vi "ExportDataToExcel.vi"(1 "DataForAnalysis":T1(array[cluster]) {"Eff" scale=0.0..30.0}, 2 "HeaderJVMetrics":string[](array[string])=["Voc (V)", "Jsc (mA/cm2)", "FF", "P (mW/cm2)", "Hyst P1/P2", "Voc (V)", "Jsc (mA/cm2)", "FF", "P (mW/cm2)", "scan rate (mV/s)", "intensity (suns)", "temperature (C)"], 3 "title":string) -> ()   [LabVIEW 2020]
uses:
  <vilib>/Utility/NIReport.llb/NI_report.lvclass
  <vilib>/addons/_office/excel.llb/Excel Easy Table (str).vi
panel:
  # "Add a title for your excel report"
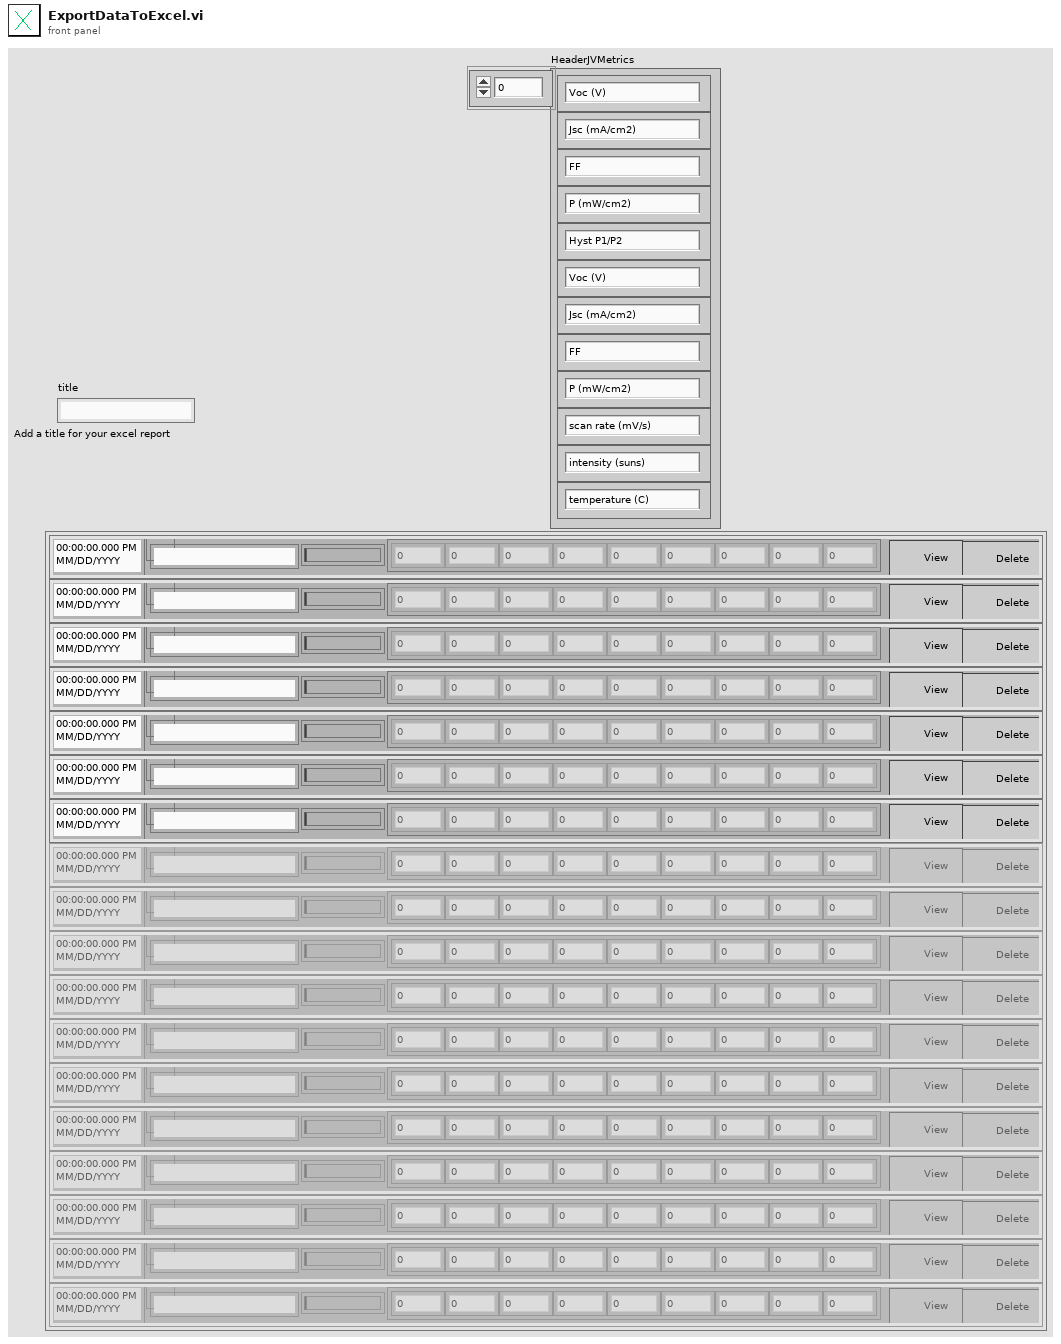
[diagram p1: front panel]
types:
  T1 = cluster{"JVData":dbl[][], "JVmetrics":dbl[], "TransientData":dbl[][], "TimeMeasured":timestamp, "Name":string, "Delete":bool, "Eff":u8, "ViewJV":bool}[]
  T2 = enum16{"Standard Report", "HTML", "Word", "Excel"}
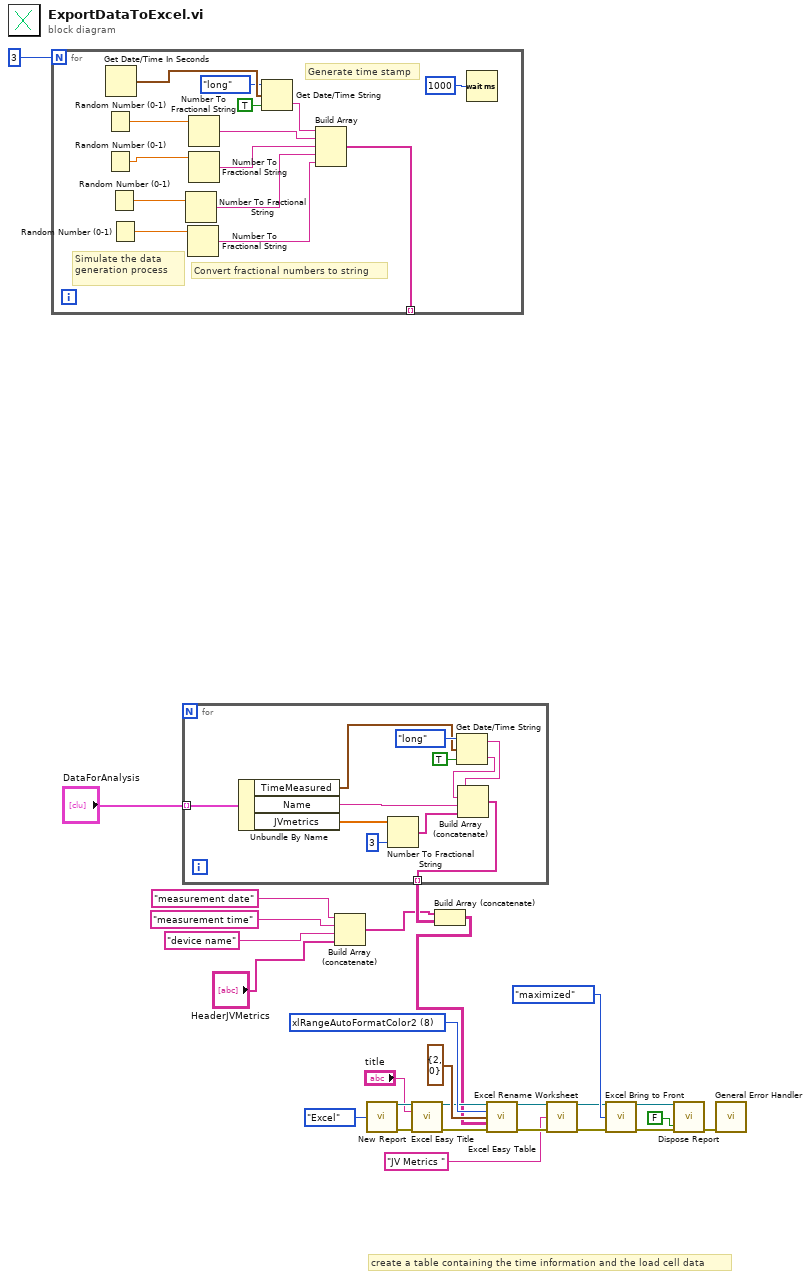
[diagram p0: block diagram]
diagram:
  w22 = 8 items=["xlRangeAutoFormat3DEffects1"=13, "xlRangeAutoFormat3DEffects2"=14, "xlRangeAutoFormatAccounting1"=4, "xlRangeAutoFormatAccounting2"=5, "xlRangeAutoFormatAccounting3"=6, "xlRangeAutoFormatAccounting4"=17, "xlRangeAutoFormatClassic1"=1, "xlRangeAutoFormatClassic2"=2, "xlRangeAutoFormatClassic3"=3, "xlRangeAutoFormatColor1"=7, "xlRangeAutoFormatColor2"=8, "xlRangeAutoFormatColor3"=9, "xlRangeAutoFormatList1"=10, "xlRangeAutoFormatList2"=11, "xlRangeAutoFormatList3"=12, "xlRangeAutoFormatLocalFormat1"=15, "xlRangeAutoFormatLocalFormat2"=16, "xlRangeAutoFormatLocalFormat3"=19, "xlRangeAutoFormatLocalFormat4"=20, "xlRangeAutoFormatReport1"=21, "xlRangeAutoFormatReport2"=22, "xlRangeAutoFormatReport3"=23, "xlRangeAutoFormatReport4"=24, "xlRangeAutoFormatReport5"=25, "xlRangeAutoFormatReport6"=26, "xlRangeAutoFormatReport7"=27, "xlRangeAutoFormatReport8"=28, "xlRangeAutoFormatReport9"=29, "xlRangeAutoFormatReport10"=30, "xlRangeAutoFormatClassicPivotTable"=31, "xlRangeAutoFormatTable1"=32, "xlRangeAutoFormatTable2"=33, "xlRangeAutoFormatTable3"=34, "xlRangeAutoFormatTable4"=35, "xlRangeAutoFormatTable5"=36, "xlRangeAutoFormatTable6"=37, "xlRangeAutoFormatTable7"=38, "xlRangeAutoFormatTable8"=39, "xlRangeAutoFormatTable9"=40, "xlRangeAutoFormatTable10"=41, "xlRangeAutoFormatPTNone"=42, "xlRangeAutoFormatNone"=-4142, "xlRangeAutoFormatSimple"=-4154] ("auto format")
  # "create a table containing the time information and the load cell data"
  n1 = for {
    N: 3 -> [_]
    tunnel: [w30] -> _ mode=indexing
    # "Convert fractional numbers to string"
    # "Generate time stamp"
    # "Simulate the data generation process"
    n2 = Random Number (0-1)() -> (number: 0 to 1=w38:dbl)
    n3 = Random Number (0-1)() -> (number: 0 to 1=w37:dbl)
    n4 = Get Date/Time In Seconds() -> (seconds since 1Jan1904=w41:timestamp)
    n5 = Random Number (0-1)() -> (number: 0 to 1=w36:dbl)
    n6 = Random Number (0-1)() -> (number: 0 to 1=w35:dbl)
    n7 = Number To Fractional String(number=w36) -> (F-format string=w32:string)  [unwired: 3 in]
    n8 = Number To Fractional String(number=w35) -> (F-format string=w31:string)  [unwired: 3 in]
    n9 = Number To Fractional String(number=w38) -> (F-format string=w34:string)  [unwired: 3 in]
    n10 = Number To Fractional String(number=w37) -> (F-format string=w33:string)  [unwired: 3 in]
    n11 = Get Date/Time String(date format (0)=enum16{"short", "long", "abbreviated"}."long", seconds (now)=w41, want seconds? (F)=TRUE) -> (time string=w28:string)  [unwired: 1 out]
    n12 = Build Array(w28, w34, w33, w32, w31) -> (w30:string[])
    n13 = Wait (ms)(milliseconds to wait=u32 1000) -> ()  [unwired: 1 out]
  }
  n14 = for {
    tunnel: "DataForAnalysis" -> [w52] mode=indexing
    tunnel: [w46] -> w12 mode=indexing
    n15 = Unbundle By Name(w52) -> ("TimeMeasured"=w47:timestamp, "Name"=w51:string, "JVmetrics"=w43:dbl[])
    n16 = Number To Fractional String(number=w43, precision (6)=i16 3) -> (F-format string=w44:string[])  [unwired: 2 in]
    n17 = Get Date/Time String(date format (0)=enum16{"short", "long", "abbreviated"}."long", seconds (now)=w47, want seconds? (F)=TRUE) -> (date string=w45:string, time string=w48:string)
    n18 = Build Array (concatenate)(w45, w48, w51, w44) -> (w46:string[])
  }
  n19 = Build Array (concatenate)("measurement date", "measurement time", "device name", "HeaderJVMetrics") -> (w8:string[])
  n20 = call <vilib>:"New Report.vi"("report type"=T2."Excel") -> ("report out"=w24:refnum<class "NI_report.lvclass">, "error out"=w25:errorcluster)  [unwired: 13 in]
  n21 = call <vilib>:"Excel Easy Title.vi"("report in"=w24, "title"="title", "error in (no error)"=w25) -> ("report out"=w16:refnum<class "NI_report.lvclass">, "error out"=w15:errorcluster)  [unwired: 10 in, 1 out]
  n22 = Build Array (concatenate)(w8, w12) -> (w7:string[][])
  n23 = call-poly <vilib>:"Excel Easy Table.vi"("report in"=w16, "auto format (none)"=w22, "start (0, 0)"=cluster{"row":i32, "column":i32} {"row"=2, "column"=0} ("position"), "text data"=w7, "error in (no error)"=w15) -> ("report out"=w5:refnum<class "NI_report.lvclass">, "error out"=w4:errorcluster)  [unwired: 6 in, 3 out]
  n24 = call <vilib>:"Excel Rename Worksheet.vi"("report in"=w5, "worksheet name (\"\")"="JV Metrics " ("string"), "error in (no error)"=w4) -> ("report out"=w3:refnum<class "NI_report.lvclass">, "error out"=w2:errorcluster)  [unwired: 11 in]
  n25 = call <vilib>:"Excel Bring to Front.vi"("report in"=w3, "window state (maximized)"=enum16{"maximized", "minimized", "normal"}."maximized", "error in (no error)"=w2) -> ("report out"=w19:refnum<class "NI_report.lvclass">, "error out"=w20:errorcluster)  [unwired: 11 in]
  n26 = call-dynamic "Dispose Report.vi"("report in"=w19, "error in (no error)"=w20, "close report? (T)"=FALSE ("Close Report? (T)")) -> ("error out"=w18:errorcluster)  [unwired: 12 in]
  n27 = call <vilib>:"General Error Handler.vi"("error in (no error)"=w18) -> ()  [unwired: 10 in, 5 out]
